vi "Clock Multiplier.vi"(6 "Enum":T1(ring)=enum."Quadrupled Frequency", 8 "Clock Gen Params":T2={"low cuttoff"=8000000.0, "high cutoff"=12000000.0, "trimmed length"=14800, "front-end samples"=400, "duty cycle (fract)"=0.6, "Gage output channel"=1}, 9 "Gage Speed":dbl(ring)=1000000000.0 items=["Slow Gage"=300000000.0, "Fast Gage"=1000000000.0], 10 "Sweep Speed":dbl=20000.0, 11 "k-space signal in":u16[](array[numeric])=array[5000 elements]) -> (3 "final waveform generated":u16[](graph))   [LabVIEW 2014]
uses:
  <vilib>/Analysis/2dsp.llb/Real FFT.vi
  <vilib>/Analysis/3filter.llb/Zero Phase Filter (obs, DBL).vi
  <vilib>/measure/maspectr.llb/FFT Power Spectrum and PSD for 1 Chan.vi
  <vilib>/measure/maresamp.llb/Resample Waveform (continuous).vi
  <vilib>/Analysis/3filter.llb/Butterworth Filter (DBL).vi
  <vilib>/Analysis/NI_AALPro.lvlib
  <vilib>/Analysis/NI_AALBase.lvlib
  <vilib>/measure/NI_MAPro.lvlib
panel:
  out "pre-upsample PSD":cluster{"f0":dbl, "df":dbl, "magnitude":dbl[]}[](graph)
  out "size(s) 2":i32
  out "upsample PSD":cluster{"f0":dbl, "df":dbl, "magnitude":dbl[]}[](graph)
  out "result":dbl
  out "Doubled Freq":dbl[](array[numeric])
  out "duty cycle (fract)":sgl=0.6
  out "Number of Points per clock sweep - 5%":dbl=47500.0
  out "No Freq Modifications":dbl[](array[numeric])
  out "low cuttoff":dbl=1000000.0
  out "high cutoff":dbl=45000000.0
  out "final waveform generated 2":dbl[][](graph)
  out "size(s)":i32=8800
  out "Freq domain (raw and filtered)":dbl[][](graph)
  out "Time domain (raw and filtered)":dbl[](graph)
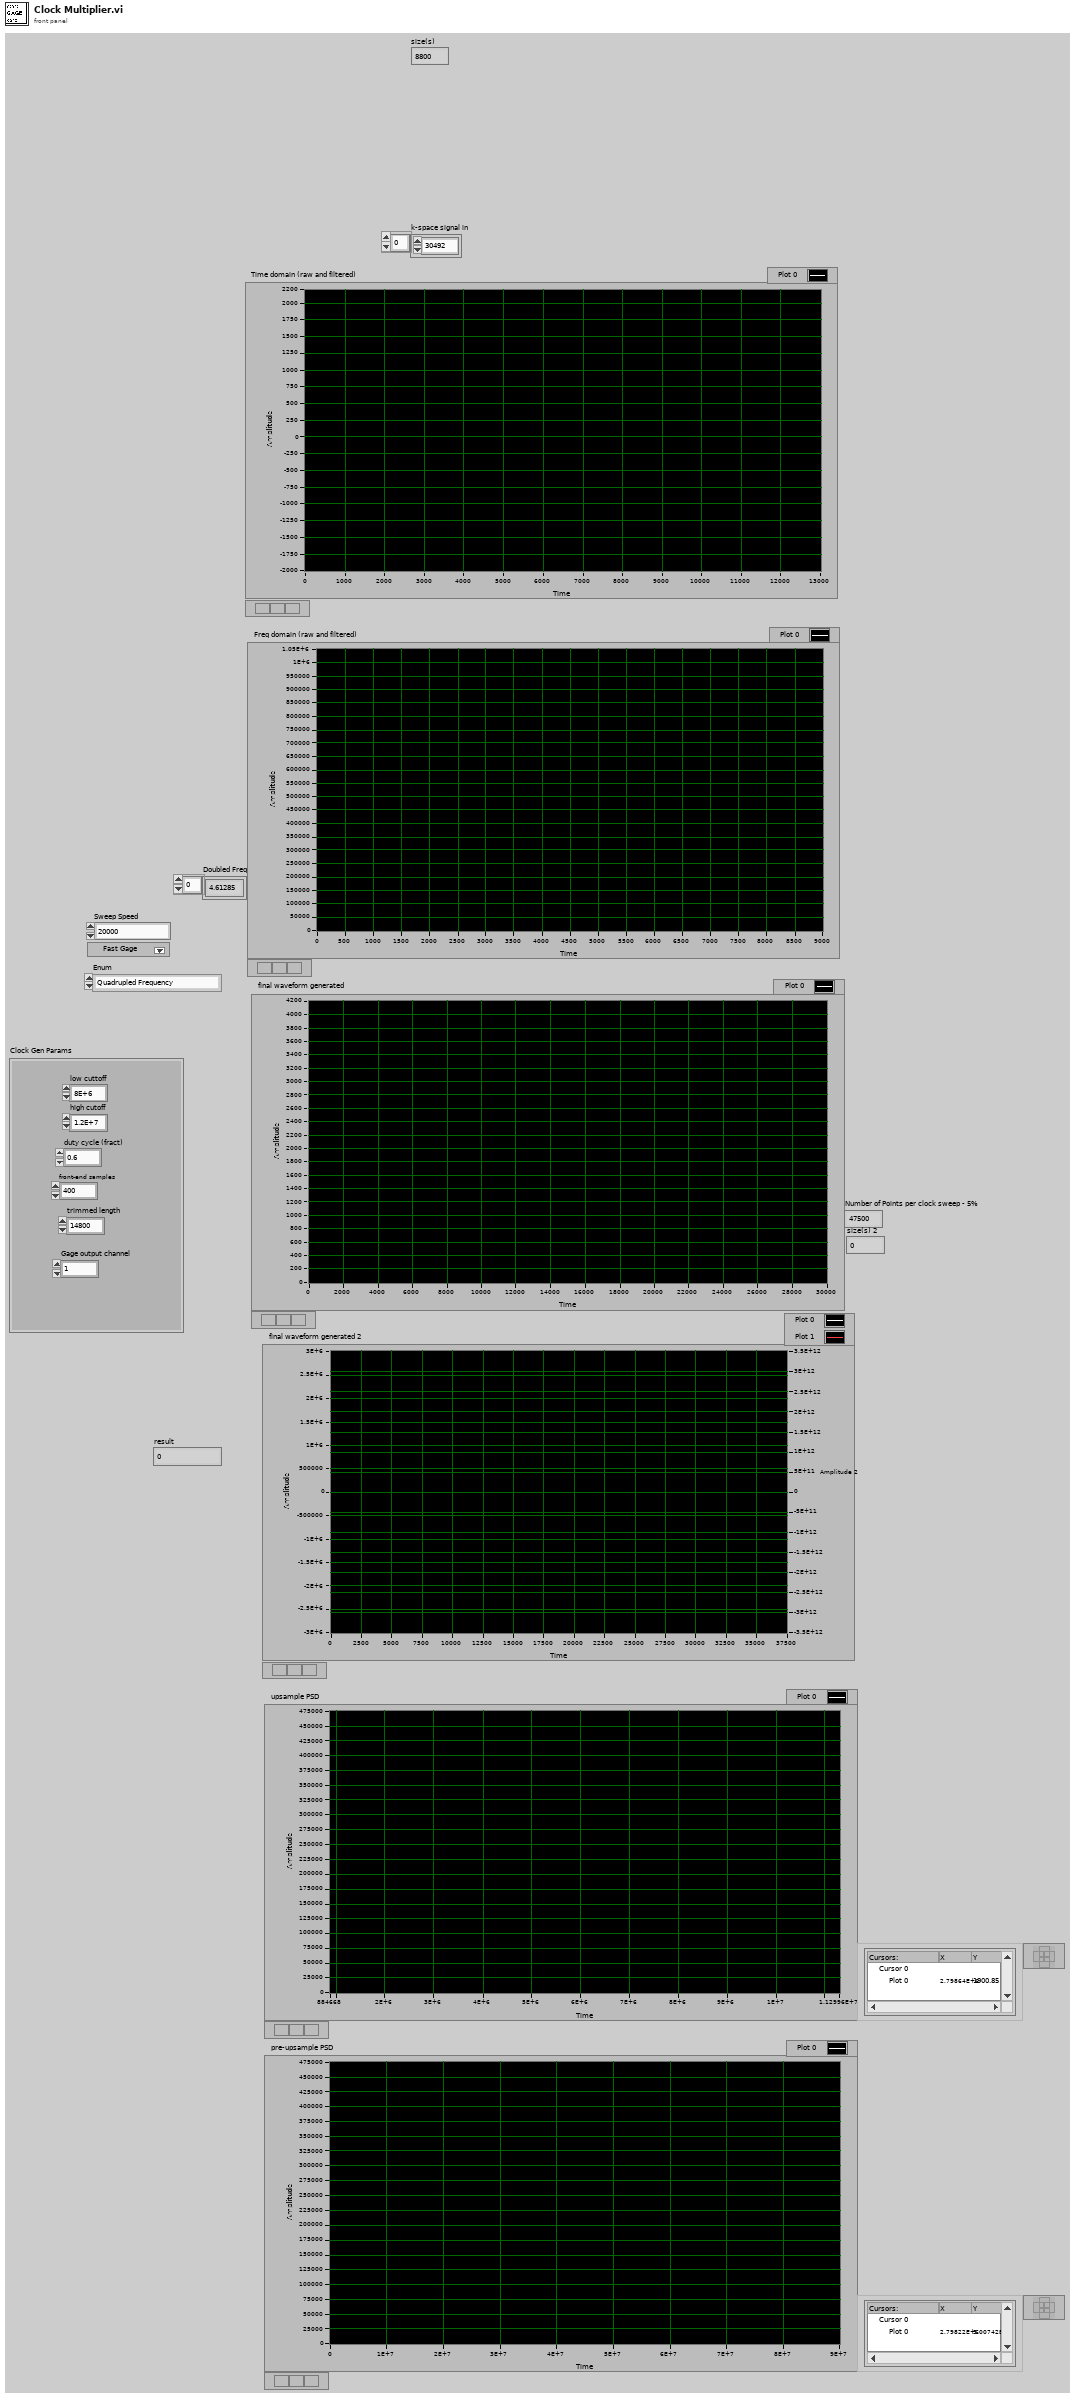
[diagram p1: front panel]
types:
  T1 = enum16{"No Frequency Enhancement", "Doubled Frequency", "Quadrupled Frequency"}
  T2 = cluster{"low cuttoff":dbl, "high cutoff":dbl, "trimmed length":i32, "front-end samples":i32, "duty cycle (fract)":sgl, "Gage output channel":i32}
  T3 = enum32{"Lowpass", "Highpass", "Bandpass", "Bandstop"}
  T4 = cluster{"filter structure":enum32{"IIR 2nd Order", "IIR 4th Order"}, "Reverse Coefficients":dbl[], "Forward Coefficients":dbl[]}
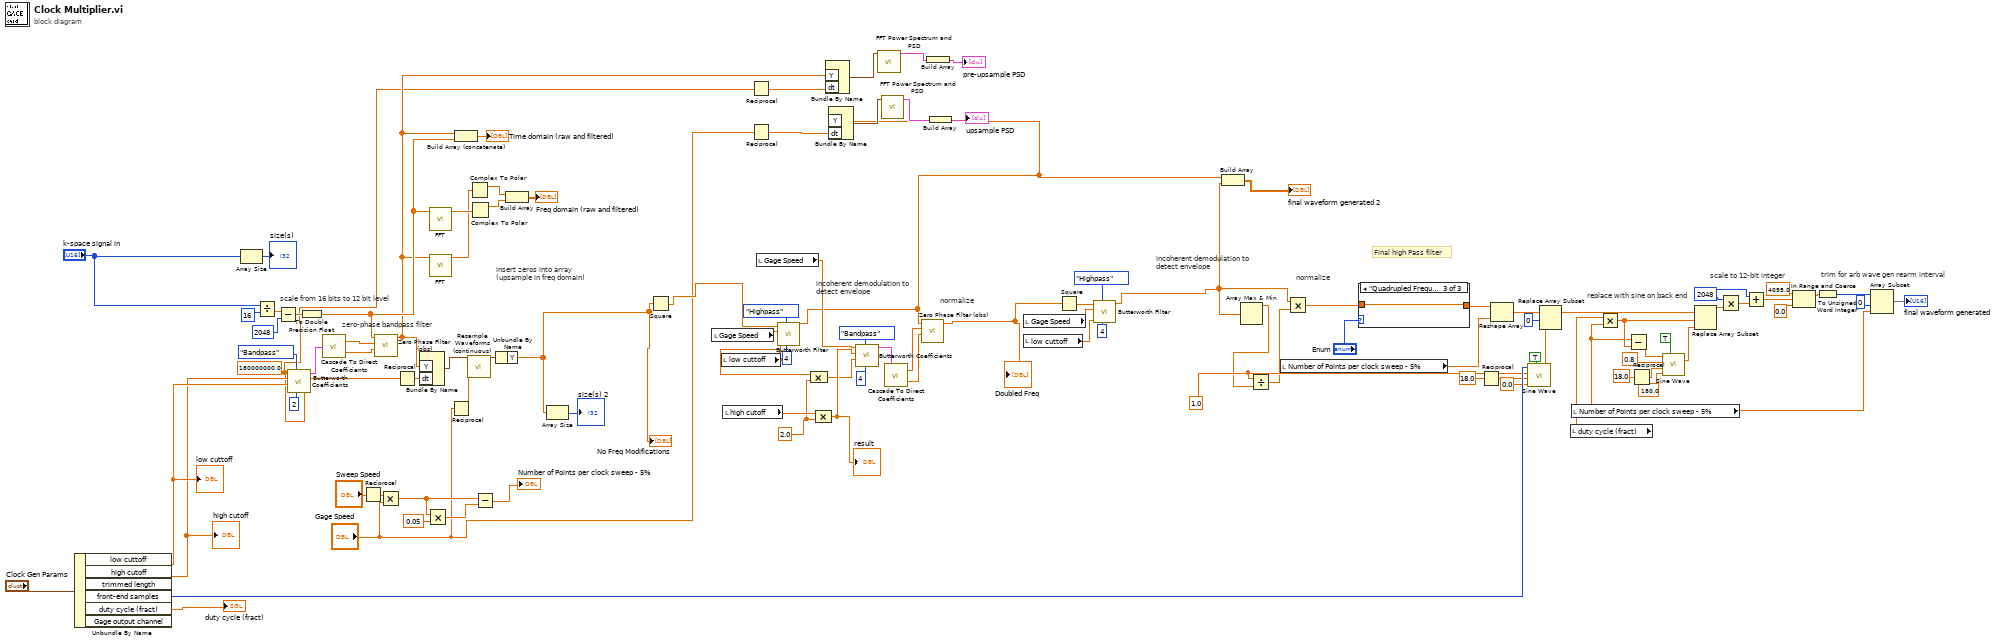
[diagram p0: block diagram]
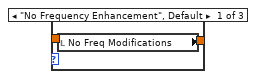
[diagram p2: hidden frame]
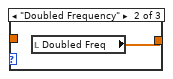
[diagram p3: hidden frame]
diagram:
  w57 = i16 2048 ("n")
  w6 = 1.0 ("amplitude")
  w29 = 2.0 ("y")
  w17 = 180000000.0 ("sampling freq: fs")
  # "trim for arb wave gen rearm interval"
  # "scale to 12-bit integer"
  # "replace with sine on back end"
  # "Final high Pass filter"
  # "normalize"
  # "incoherent demodulation to\ndetect envelope"
  # "normalize"
  # "incoherent demodulation to\ndetect envelope"
  # "scale from 16 bits to 12 bit level"
  # "insert zeros into array\n(upsample in freq domain)"
  # "zero-phase bandpass filter"
  n1 = Unbundle By Name("Clock Gen Params") -> ("low cuttoff"=w80:dbl, "high cutoff"=w79:dbl, "front-end samples"=w91:i32, "duty cycle (fract)"=→"duty cycle (fract)":sgl)  [unwired: 2 out]
  "high cutoff" <- w79
  "low cuttoff" <- w80
  n2 = Array Size(array="k-space signal in") -> (size(s)=→"size(s)":i32)
  n3 = Divide(x="k-space signal in", y=i16 16 ("n")) -> (x/y=w103:dbl[])
  n4 = Subtract(x=w103, y=i16 2048 ("n")) -> (x-y=w93:dbl[])
  n5 = call <vilib>:"Butterworth Coefficients.vi"("order"=2, "filter type"=T3."Bandpass", "low cutoff freq: fl"=w80, "high cutoff freq: fh"=w79, "sampling freq: fs"=w17) -> ("IIR Filter Cluster"=w42:T4)  [unwired: 5 in, 1 out]
  n6 = To Double Precision Float(number=w93) -> (double precision float=w39:dbl[])
  n7 = call <vilib>:"Cascade To Direct Coefficients.vi"("IIR Filter Cluster"=w42) -> ("Reverse Coefficients"=w41:dbl[], "Forward Coefficients"=w40:dbl[])
  n8 = Reciprocal(x="Sweep Speed") -> (1/x=w85:dbl)
  n9 = call-poly <vilib>:"Zero Phase Filter (obs).vi"("Forward Coefficients"=w40, "Reverse Coefficients"=w41, "X"=w39) -> ("Filtered X"=w18:dbl[])  [unwired: 7 in, 1 out]
  n10 = Multiply(x=w85, y="Gage Speed") -> (x*y=w19:dbl)
  n11 = Reciprocal(x=w17) -> (1/x=w16:dbl)
  n12 = Bundle By Name("Y"=w18, "dt"=w16) -> (w15:waveform(dbl))  [unwired: 1 in]
  n13 = Multiply(x=w19, y=0.05) -> (x*y=w81:dbl)
  n14 = call-poly <vilib>:"FFT.vi"("X"=w39) -> ("FFT {X}"=w94:cdb[])  [unwired: 9 in, 1 out]
  n15 = call-poly <vilib>:"FFT.vi"("X"=w18) -> ("FFT {X}"=w20:cdb[])  [unwired: 9 in, 1 out]
  n16 = Reciprocal(x="Gage Speed") -> (1/x=w13:dbl)
  n17 = Build Array (concatenate)(w18, w39) -> (→"Time domain (raw and filtered)":dbl[])
  n18 = call-poly <vilib>:"Resample Waveforms (continuous).vi"("waveform in"=w15, "dt"=w13) -> ("resampled waveform out"=w12:waveform(dbl))  [unwired: 9 in, 4 out]
  n19 = Complex To Polar(r * e^(i*theta)=w20) -> (r=w100:dbl[])  [unwired: 1 out]
  n20 = Complex To Polar(r * e^(i*theta)=w94) -> (r=w101:dbl[])  [unwired: 1 out]
  n21 = Subtract(x=w19, y=w81) -> (x-y=→"Number of Points per clock sweep - 5%":dbl)
  n22 = Unbundle By Name(w12) -> ("Y"=w10:dbl[])
  "No Freq Modifications" <- w10
  n23 = Build Array(w100, w101) -> (→"Freq domain (raw and filtered)":dbl[][])
  n24 = Array Size(array=w10) -> (size(s)=→"size(s) 2":i32)
  n25 = Square(x=w10) -> (x^2=w27:dbl[])
  n26 = local read "Gage Speed"() -> (w78:dbl)
  n27 = local read "low cuttoff"() -> (w30:dbl)
  n28 = local read "high cutoff"() -> (w33:dbl)
  n29 = Reciprocal(x=w17) -> (1/x=w24:dbl)
  n30 = Reciprocal(x="Gage Speed") -> (1/x=w34:dbl)
  n31 = local read "Gage Speed"() -> (w77:dbl)
  n32 = call-poly <vilib>:"Butterworth Filter.vi"("order"=4, "filter type"=T3."Highpass", "low cutoff freq: fl"=w30, "sampling freq: fs"=w78, "X"=w27) -> ("Filtered X"=w9:dbl[])  [unwired: 3 in, 1 out]
  n33 = Compound Arithmetic op=MULTIPLY(w30, w29) -> (w28:dbl)
  n34 = Compound Arithmetic op=MULTIPLY(w33, w29) -> (w31:dbl)
  "result" <- w31
  n35 = Bundle By Name("Y"=w18, "dt"=w24) -> (w25:waveform(dbl))  [unwired: 1 in]
  n36 = Bundle By Name("Y"=w9, "dt"=w34) -> (w11:waveform(dbl))  [unwired: 1 in]
  n37 = call <vilib>:"Butterworth Coefficients.vi"("order"=4, "filter type"=T3."Bandpass", "low cutoff freq: fl"=w28, "high cutoff freq: fh"=w31, "sampling freq: fs"=w77) -> ("IIR Filter Cluster"=w38:T4)  [unwired: 5 in, 1 out]
  n38 = call-poly <vilib>:"FFT Power Spectrum and PSD.vi"("time signal"=w25) -> ("Power Spectrum / PSD"=w22:cluster{"f0":dbl, "df":dbl, "magnitude":dbl[]})  [unwired: 7 in, 3 out]
  n39 = call-poly <vilib>:"FFT Power Spectrum and PSD.vi"("time signal"=w11) -> ("Power Spectrum / PSD"=w23:cluster{"f0":dbl, "df":dbl, "magnitude":dbl[]})  [unwired: 7 in, 3 out]
  n40 = call <vilib>:"Cascade To Direct Coefficients.vi"("IIR Filter Cluster"=w38) -> ("Reverse Coefficients"=w37:dbl[], "Forward Coefficients"=w36:dbl[])
  n41 = call-poly <vilib>:"Zero Phase Filter (obs).vi"("Forward Coefficients"=w36, "Reverse Coefficients"=w37, "X"=w9) -> ("Filtered X"=w8:dbl[])  [unwired: 7 in, 1 out]
  "Doubled Freq" <- w8
  n42 = Build Array(w22) -> (→"pre-upsample PSD":cluster{"f0":dbl, "df":dbl, "magnitude":dbl[]}[])
  n43 = Build Array(w23) -> (→"upsample PSD":cluster{"f0":dbl, "df":dbl, "magnitude":dbl[]}[])
  n44 = local read "Gage Speed"() -> (w75:dbl)
  n45 = local read "low cuttoff"() -> (w74:dbl)
  n46 = Square(x=w8) -> (x^2=w7:dbl[])
  n47 = call-poly <vilib>:"Butterworth Filter.vi"("order"=4, "filter type"=T3."Highpass", "low cutoff freq: fl"=w74, "sampling freq: fs"=w75, "X"=w7) -> ("Filtered X"=w3:dbl[])  [unwired: 3 in, 1 out]
  n48 = Build Array(w9, w3) -> (→"final waveform generated 2":dbl[][])
  n49 = Array Max & Min(array=w3) -> (max value=w5:dbl)  [unwired: 3 out]
  n50 = Divide(x=w6, y=w5) -> (x/y=w4:dbl)
  n51 = local read "Number of Points per clock sweep - 5%"() -> (w47:dbl)
  n52 = Multiply(x=w3, y=w4) -> (x*y=w2:dbl[])
  n53 = case shown="\"Quadrupled Frequency\"" "Enum" {
    tunnel: [w106 w107 w108] -> w45
    tunnel: w2 -> [_ _ w108]
    frame "No Frequency Enhancement", Default {
      n54 = local read "No Freq Modifications"() -> (w106:dbl[])
    }
    frame "Doubled Frequency" {
      n55 = local read "Doubled Freq"() -> (w107:dbl[])
    }
    frame "Quadrupled Frequency" {
    }
  }
  n56 = Reciprocal(x=18.0 ("amplitude")) -> (1/x=w67:dbl)
  n57 = Reshape Array(w45, w47) -> (w46:dbl[])
  n58 = call <vilib>:"Sine Wave.vi"("samples"=w91, "amplitude"=w6, "frequency"=w67, "phase in"=0.0, "reset phase"=TRUE) -> ("sine wave"=w68:dbl[])  [unwired: 2 out]
  n59 = Replace Array Subset(array=w46, new element=w68, index=0) -> (w60:dbl[])
  n60 = local read "duty cycle (fract)"() -> (w43:sgl)
  n61 = local read "Number of Points per clock sweep - 5%"() -> (w44:dbl)
  n62 = Multiply(x=w43, y=w44) -> (x*y=w52:dbl)
  n63 = Subtract(x=w44, y=w52) -> (x-y=w53:dbl)
  n64 = Reciprocal(x=18.0 ("amplitude")) -> (1/x=w64:dbl)
  n65 = call <vilib>:"Sine Wave.vi"("samples"=w53, "amplitude"=0.8, "frequency"=w64, "phase in"=180.0, "reset phase"=TRUE) -> ("sine wave"=w59:dbl[])  [unwired: 2 out]
  n66 = Replace Array Subset(array=w60, new element=w59, index=w52) -> (w48:dbl[])
  n67 = Multiply(x=w57, y=w48) -> (x*y=w58:dbl[])
  n68 = Add(x=w57, y=w58) -> (x+y=w49:dbl[])
  n69 = In Range and Coerce(upper limit=sgl 4095.0 ("n"), x=w49, lower limit=sgl 0.0 ("n")) -> (coerced(x)=w50:dbl[])  [unwired: 1 out]
  n70 = To Unsigned Word Integer(number=w50) -> (unsigned 16bit integer=w56:u16[])
  n71 = Array Subset(array=w56, index=0, length=w44) -> (→"final waveform generated":u16[])
